vi "EnableLoopBack.vi"(10 "Enable Loopback":u64, 11 "Reference ID":u64) -> (0 "Error code":i32, 3 "Reference ID out":u64)   [LabVIEW 2023]
doc: "Enables loop back by turning on Loop back boolean"
uses:
  <vilib>/Utility/error.llb/Error Cluster From Error Code.vi
  <vilib>/rvi/errors/niLvFpgaAdjustHostInterfaceError.vi
  <vilib>/rvi/interface/nirviReadWriteControl/nirviReadWriteControl.xnode
  NiFpgaLv.dll
  <vilib>/rvi/interface/Simulation/niFpgaSimulationCallBeginRW.vi
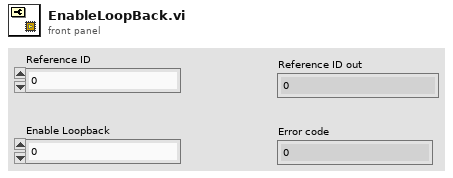
[diagram p1: front panel]
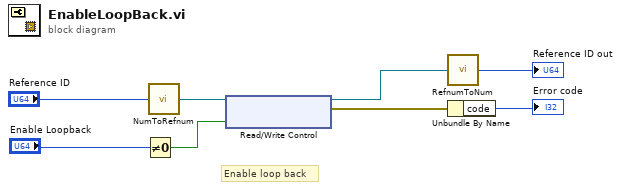
[diagram p0: block diagram]
diagram:
  # "Enable loop back"
  n1 = Not Equal To 0?(x="Enable Loopback") -> (x != 0?=w1:bool)
  n2 = call "NumToRefnum.vi"("Reference ID"="Reference ID") -> ("Refnum Out"=w8:refnum<k20>)
  n3 = xnode ("Read/Write Control")("FPGA VI Reference In"=w8, "EnableLoopBack"=w1) -> ("FPGA VI Reference Out"=w7:refnum<k20>, "error out"=w4:errorcluster)  [unwired: 1 in]
  n4 = call "RefnumToNum.vi"("Refnum in"=w7) -> ("Reference ID"=→"Reference ID out":u64)
  n5 = Unbundle By Name(w4) -> ("code"=→"Error code":i32)
